vi "Aperture Cal2.vi"(0 "Red BCG Values (Brightness 1)":T5={"Brightness"=128.0, "Contrast"=45.0, "Gamma"=1.0}, 1 "Green BCG Values (Brightness 1)":T5={"Brightness"=128.0, "Contrast"=45.0, "Gamma"=1.0}, 2 "Blue BCG Values (Brightness 1)":T5={"Brightness"=128.0, "Contrast"=45.0, "Gamma"=1.0}, 3 "Grid Descriptor (Aperture Calibration)":T3={"X Step"=6.25, "Y Step"=6.25, "Unit"=enum."Micrometer"} {"Y Step" format="%.2f"; "X Step" format="%.2f"}, 4 "Calibration Axis Info (Aperture Calibration)":T2={"Origin Pixel"={"X"=227.0, "Y"=1000.0}, "X Axis Pixel"={"X"=276.9972, "Y"=1000.52985}, "Axis Reference"=1} {"Axis Reference" items=["Direct", "Indirect"]}, 5 "ROI Descriptor (Line)":T1={"Global Rectangle"=[88, 1000, 713, 1001], "Contours"=[{"ID"=enum."External", "Type"=2, "Coordinates"=[88, 1000, 712, 1000]}]} {"Contours"."Type" items=["No Selection", "Point", "Line", "Rectangle", "Oval", "Polygon", "Freehand Region", "Annulus", "Unused2", "Unused3", "Broken Line", "Freehand Line", "Rotated Rectangle"]}, 7 "error in":errorcluster) -> (20 "Line Profile (Line)":u8[][](array[numeric]), 27 "error out":errorcluster)   [LabVIEW 2018]
uses:
  <vilib>/vision/Image Controls.llb/Vision Info Type2.ctl
  <vilib>/vision/NI_Vision_Development_Module.lvlib
panel:
  out "Image Out":T6(plugin-control)
  out "Line Profile Graph":u8[][](graph) caption="Line Profile"
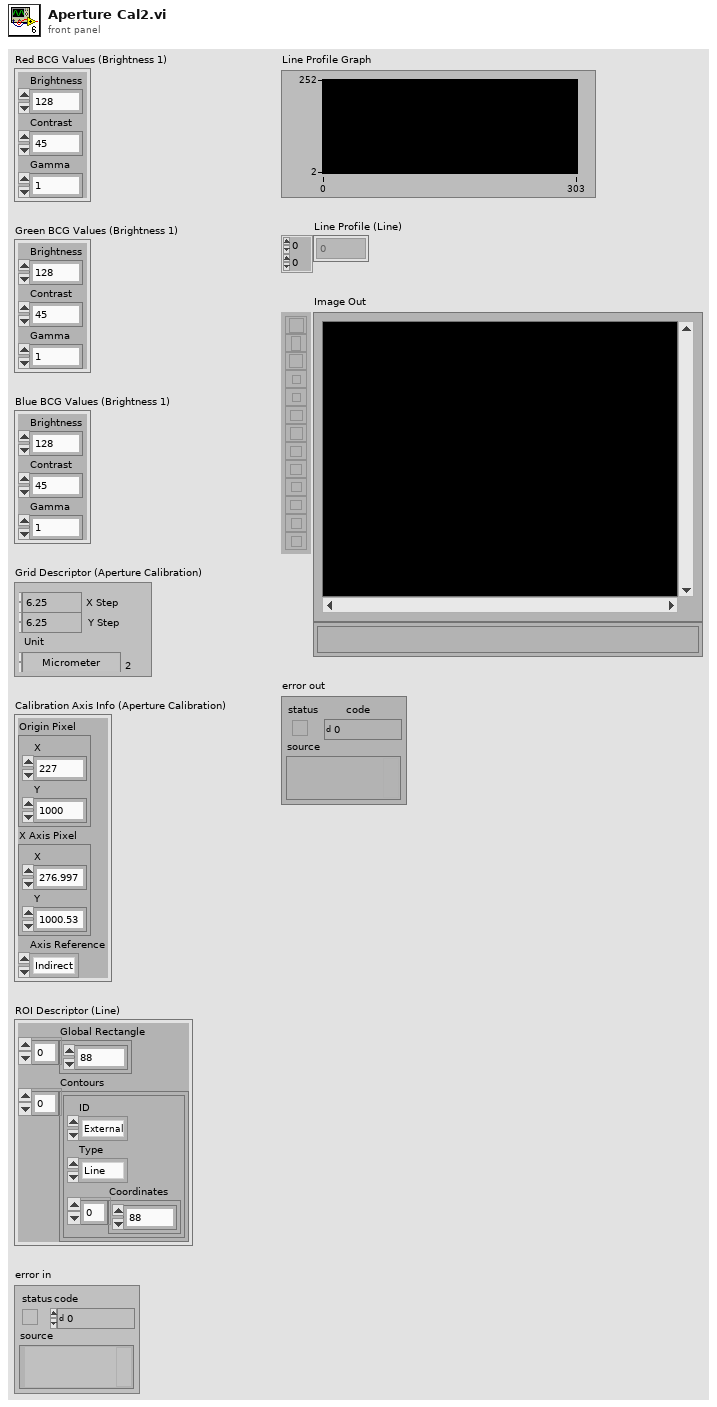
[diagram p1: front panel]
types:
  T1 = cluster{"Global Rectangle":i32[], "Contours":cluster{"ID":enum32{"External", "Internal"}, "Type":u32, "Coordinates":i32[]}[]}
  T2 = cluster{"Origin Pixel":cluster{"X":sgl, "Y":sgl}, "X Axis Pixel":cluster{"X":sgl, "Y":sgl}, "Axis Reference":u32}
  T3 = typedef "Simple Grid Descriptor" = cluster{"X Step":sgl, "Y Step":sgl, "Unit":T4}
  T4 = typedef "Image Unit" = enum32{"Undefined", "Angström", "Micrometer", "Millimeter", "Centimeter", "Meter", "Kilometer", "Microinch", "Inch", "Feet", "Nautical miles", "Standard miles", "Steps"}
  T5 = cluster{"Brightness":sgl, "Contrast":sgl, "Gamma":sgl}
  T6 = typedef "IMAQ Image.ctl" = refnum<image>
  T7 = typedef "Vision Info Type2.ctl" = u32
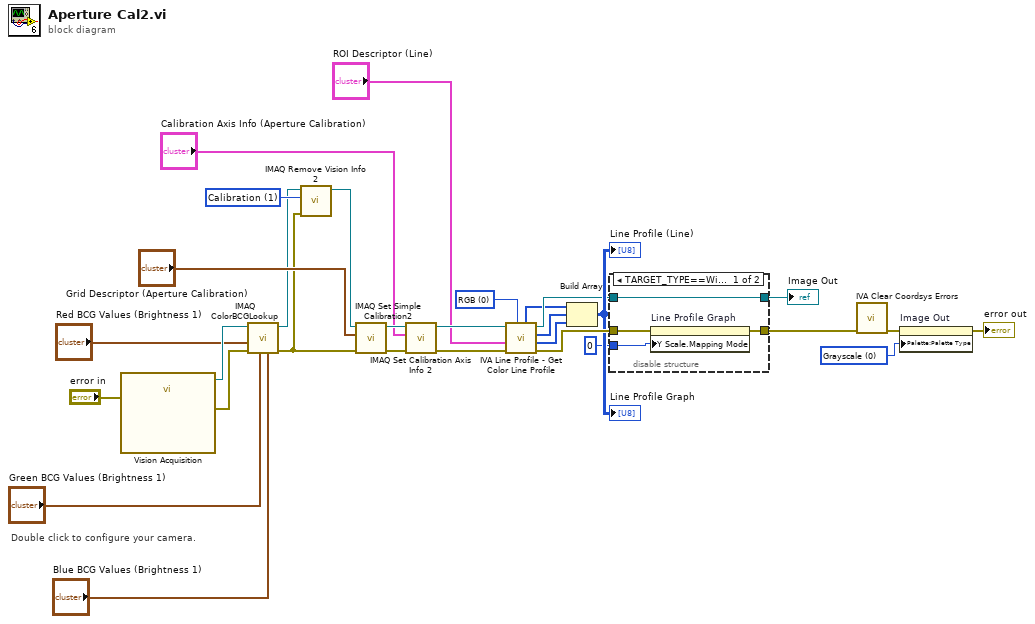
[diagram p0: block diagram]
diagram:
  w1 = u32 0 items=["Grayscale", "Binary", "Gradient", "Rainbow", "Temperature", "User Defined", "Binary 16 Bit", "Gradient 16 Bit", "Rainbow 16 Bit", "Temperature 16 Bit", "User Defined 16 Bit"] ("Palette Type")
  w15 = u16 0 items=["RGB", "HSL", "HSV", "HSI"] ("Color Mode")
  w23 = T7 1 items=["Any", "Calibration", "Overlay", "Grayscale Template", "Color Template", "Geometric Template", "Custom Data", "Golden Template", "Geometric Template 2", "Contour Data", "Camera Model"] ("Vision Info")
  # "Double click to configure your camera."
  n1 = call "Vision Acquisition"("error in"="error in") -> ("Image Out"=w29:T6, "error out"=w28:errorcluster)  [unwired: 25 in]
  n2 = call "IMAQ ColorBCGLookup"("Blue BCG Values"="Blue BCG Values (Brightness 1)", "Green BCG Values"="Green BCG Values (Brightness 1)", "error in (no error)"=w28, "Red BCG Values"="Red BCG Values (Brightness 1)", "Image Src"=w29) -> ("error out"=w20:errorcluster, "Image Dst Out"=w22:T6)  [unwired: 2 in, 3 out]
  n3 = call "IMAQ Remove Vision Info 2"("error in (no error)"=w20, "Vision Info"=w23, "Image"=w22) -> ("Image Out"=w21:T6)  [unwired: 8 out]
  n4 = call "IMAQ Set Simple Calibration2"("error in (no error)"=w20, "Pixel Distances"="Grid Descriptor (Aperture Calibration)", "Image"=w21) -> ("error out"=w18:errorcluster, "Calibration Template Image"=w19:T6)  [unwired: 2 in, 5 out]
  n5 = call-poly "IMAQ Set Calibration Axis Info 2"("error in (no error)"=w18, "Calibration Axis Info"="Calibration Axis Info (Aperture Calibration)", "Calibration Template Image In"=w19) -> ("error out"=w11:errorcluster, "Calibration Template Image Out"=w14:T6)  [unwired: 7 out]
  n6 = call <vilib>:"IVA Line Profile - Get Color Line Profile.vi"("Color Mode"=w15, "error in (no error)"=w11, "ROI Descriptor"="ROI Descriptor (Line)", "Image In"=w14) -> ("error out"=w16:errorcluster, "Blue or Luma Pixels"=w6:u8[], "Green or Sat Pixels"=w7:u8[], "Image Out"=w10:T6, "Red or Hue Pixels"=w8:u8[])  [unwired: 3 out]
  n7 = Build Array(w8, w7, w6) -> (→"Line Profile Graph" →"Line Profile (Line)":u8[][])
  n8 = disable-structure "Conditional Disable Structure" shown="TARGET_TYPE==Windows" {
    disable-tunnel: w16 -> [w34 w35]
    disable-tunnel: [w33 w35] -> w5
    disable-tunnel: w10 -> [w32 w36]
    disable-tunnel: [w32 w36] -> w2
    disable-tunnel: u8 0 ("Y Scale.Mapping Mode") -> [w31 _]
    frame condition #0 (active) {
      n9 = property on="Line Profile Graph" class="WFGraph (strict)"(error in=w34, "Y Scale.Mapping Mode"=w31) -> (error out=w33:errorcluster)  [unwired: 1 in, 1 out]
    }
    frame condition #1 {
    }
  }
  "Image Out" <- w2
  n10 = call <vilib>:"IVA Clear Coordsys Errors.vi"("error in (no error)"=w5) -> ("error out"=w4:errorcluster)  [unwired: 10 in]
  n11 = property on="Image Out" class="ImageControl"(error in=w4, "Palette:Palette Type"=w1) -> (error out=→"error out":errorcluster)  [unwired: 1 in, 1 out]
